vi "GetSEQHZOffset.vi"(4 "2ND Source (1: Channel 2)":u16(ring)=1 items=["Channel 1", "Channel 2", "Channel 3", "Channel 4"], 5 "2nd Channel?":bool=TRUE, 6 "error in (no error)":errorcluster, 8 "1ST Source (0: Channel 1)":u16(ring) items=["Channel 1", "Channel 2", "Channel 3", "Channel 4"], 9 "VISA resource name":refnum<visa-resource-name>="HDO6104") -> (0 "error out":errorcluster, 1 "Run Time (s)":sgl, 2 "CH2 HZ OFFSET":dbl[](array[numeric]), 3 "CH1 HZ OFFSET":dbl[](array[numeric]))   [LabVIEW 2022 SP3]
uses:
  <instrlib>/LeCroy Wave Series/LeCroy Wave Series.lvlib
panel:
  out "Array":dbl[](array[numeric])
  out "Waveform Graph 2":dbl[](graph)
  out "Waveform Graph":dbl[](graph)
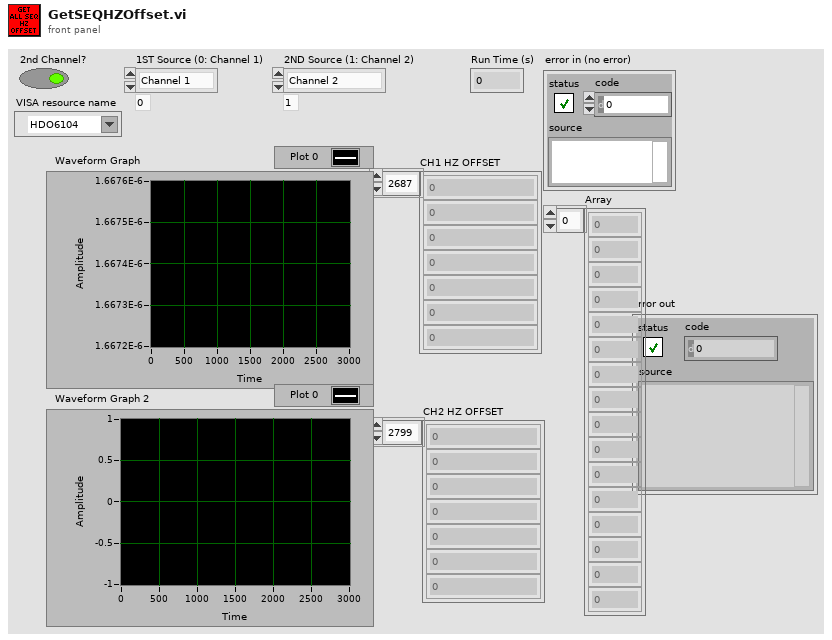
[diagram p1: front panel]
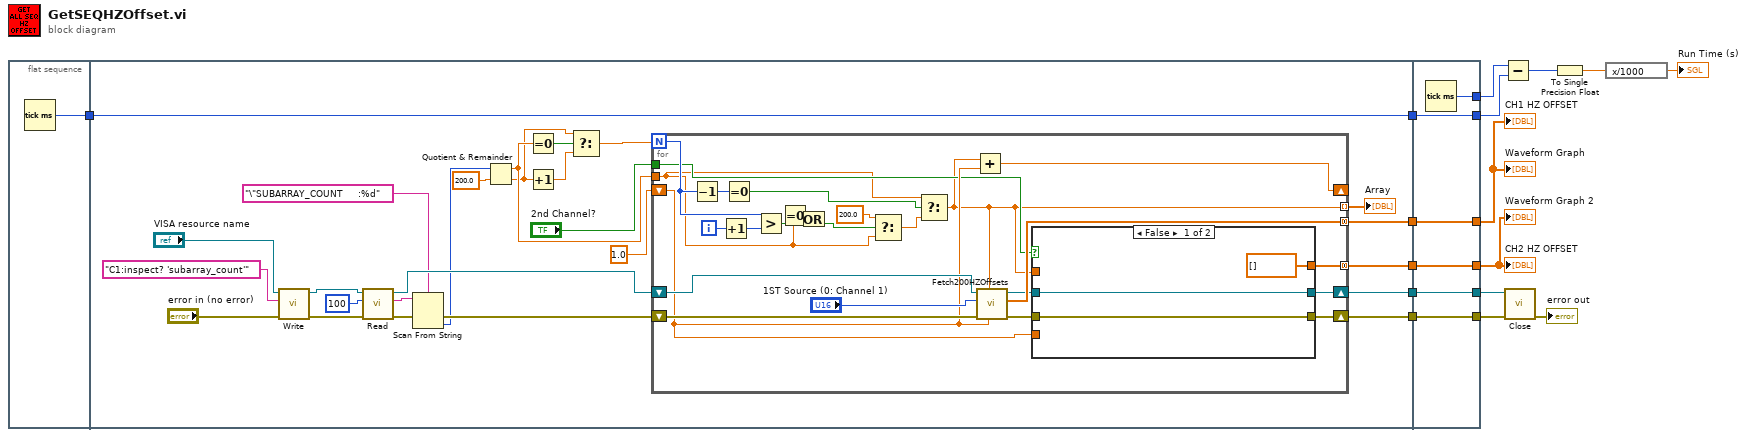
[diagram p0: block diagram]
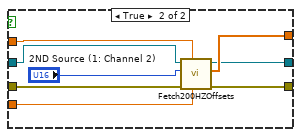
[diagram p2: hidden frame]
diagram:
  n1 = flat-sequence {
    tunnel: [w17] -> w11
    tunnel: w11 -> [w19]
    tunnel: [w42] -> w6
    tunnel: [w41] -> w5
    tunnel: [w40] -> w4
    tunnel: [w39] -> w3
    tunnel: [w19] -> w2
    tunnel: [w80] -> w10
    tunnel: [w81] -> w12
    tunnel: [w82] -> w13
    tunnel: [w83] -> w14
    tunnel: [w84] -> w15
    tunnel: w6 -> [w84]
    tunnel: w5 -> [w83]
    tunnel: w4 -> [w82]
    tunnel: w3 -> [w81]
    tunnel: w2 -> [w80]
    tunnel: [w79] -> w1
    frame #0 {
      n2 = Tick Count (ms)() -> (millisecond timer value=w17:u32)
    }
    frame #1 {
      n3 = call <instrlib>:"Write.vi"("error in (no error)"="error in (no error)", "Write Buffer"="C1:inspect? 'subarray_count'", "VISA resource name"="VISA resource name") -> ("error out"=w37:errorcluster, "VISA resource name out"=w38:refnum<visa-resource-name>)  [unwired: 6 in, 1 out]
      n4 = call <instrlib>:"Read.vi"("error in (no error)"=w37, "Byte Count"=u32 100, "VISA resource name"=w38) -> ("error out"=w34:errorcluster, "Read Buffer"=w35:string, "VISA resource name out"=w33:refnum<visa-resource-name>)  [unwired: 5 in, 1 out]
      n5 = Scan From String(format string="\"SUBARRAY_COUNT     :%d", input string=w35, error in=w34) -> (error out=w32:errorcluster, output 1=w28:i32)  [unwired: 2 in, 2 out]
      n6 = Quotient & Remainder(x=w28, y=200.0) -> (x-y*floor(x/y)=w27:dbl, floor(x/y)=w24:dbl)
      n7 = Equal To 0?(x=w27) -> (x = 0?=w26:bool)
      n8 = Increment(x=w24) -> (x+1=w25:dbl)
      n9 = Select(t=w24, s=w26, f=w25) -> (s? t:f=w23:dbl)
      n10 = for {
        N: w23 -> [w63]
        tunnel: [w67] -> w40 mode=concatenating
        tunnel: [w50] -> w39 mode=concatenating
        shift-right: [w49] -> w42
        shift-left: w33 -> [w56]
        shift-right: [w51] -> w41
        shift-left: w32 -> [w66]
        tunnel: w27 -> [w45]
        shift-right: [w57] -> _
        shift-left: 1.0 ("y") -> [w53]
        tunnel: "2nd Channel?" -> [w48]
        tunnel: [w47] -> w18 mode=indexing
        i -> [w58]
        n11 = Decrement(x=w63) -> (x-1=w61:i32)
        n12 = Increment(x=w58) -> (x+1=w59:i32)
        n13 = Equal To 0?(x=w61) -> (x = 0?=w62:bool)
        n14 = Greater?(x=w63, y=w59) -> (0:w64:bool)
        n15 = Equal To 0?(x=w45) -> (x = 0?=w44:bool)
        n16 = Or(x=w44, y=w64) -> (x .or. y?=w46:bool)
        n17 = Select(t=200.0, s=w46, f=w45) -> (s? t:f=w60:dbl)
        n18 = Select(t=w45, s=w62, f=w60) -> (s? t:f=w47:dbl)
        n19 = Add(x=w47, y=w53) -> (x+y=w57:dbl)
        n20 = call "Fetch200HZOffsets.vi"("First Segment"=w53, "Number of Segments"=w47, "error in (no error)"=w66, "Source (0: Channel 1)"="1ST Source (0: Channel 1)", "VISA Resource Name in"=w56) -> ("error out"=w52:errorcluster, "HZ offsets"=w67:dbl[], "VISA Resource Name out"=w54:refnum<visa-resource-name>)  [unwired: 4 in]
        n21 = case shown="False" w48 {
          tunnel: w54 -> [w69 w78]
          tunnel: w47 -> [_ w77]
          tunnel: w53 -> [_ w76]
          tunnel: w52 -> [w68 w75]
          tunnel: [w68 w74] -> w51
          tunnel: [dbl[] [] ("HZ offsets") w73] -> w50
          tunnel: [w69 w72] -> w49
          frame False {
          }
          frame True {
            n22 = call "Fetch200HZOffsets.vi"("First Segment"=w76, "Number of Segments"=w77, "error in (no error)"=w75, "Source (0: Channel 1)"="2ND Source (1: Channel 2)", "VISA Resource Name in"=w78) -> ("error out"=w74:errorcluster, "HZ offsets"=w73:dbl[], "VISA Resource Name out"=w72:refnum<visa-resource-name>)  [unwired: 4 in]
          }
        }
      }
      "Array" <- w18
    }
    frame #2 {
      n23 = Tick Count (ms)() -> (millisecond timer value=w79:u32)
    }
  }
  n24 = Subtract(x=w1, y=w10) -> (x-y=w9:u32)
  n25 = call <instrlib>:"Close.vi"("error in (no error)"=w14, "VISA resource name"=w15) -> ("error out"=→"error out":errorcluster)  [unwired: 9 in]
  n26 = To Single Precision Float(number=w9) -> (single precision float=w7:sgl)
  n27 = expression code="x/1000"(w7) -> (→"Run Time (s)":sgl)
  "CH1 HZ OFFSET" <- w13
  "Waveform Graph" <- w13
  "CH2 HZ OFFSET" <- w12
  "Waveform Graph 2" <- w12
